vi "Main.vi"() -> ()   [LabVIEW 2025]
uses:
  State.ctl
  Replacement Channels.ctl
  NationalInstruments.VeriStand.SystemDefinitionAPI
panel:
  out "Array":T1[](array[typedef])
  out "Numeric":i32
  out "Deleted Channels":string[](array[string])
  in  "Delete Deprecated Channels":bool
  out "State":T2
  out "Replacement Log":string[](array[string])
  in  "stop":bool
  in  "Replace Signals":bool
  in  "Run Comparison Utility":bool
  in  "Available VCOM Signals (Replacement Channels)":string[](array[combo])=["CAN_Sender_Rx.ACC.ACC_ESP_E2E_PR2.ACC_ESP_E2E_PR2_CRC", "ESP_Rx.ACC.ACC_ESP_E2E_PR2.ACC_ESP_E2E_PR2_CRC", "CAN_Sender_Tx.ACC.NM_ACC.NM_ACC_ID", "ESP_Tx.ACC.NM_ACC.NM_ACC_ID"]
  in  "System Definition File Path":path=path "C:/dev/VCOM-SysDef-Utility/VCOM Config System Definition Utility/VeriStand Example Project/Example Project/Example Project.nivssdf"
  in  "Error in":errorcluster
  out "Signals Not Found in new VCOM Config (Channels to Replace)":string[](array[string])
  out "error out":errorcluster
  in  "VCOM config file in":path=path "C:/Users/Public/Documents/National Instruments/NI-VCOM/configuration/Single_Point/CAN/VCOMConfig.xml"
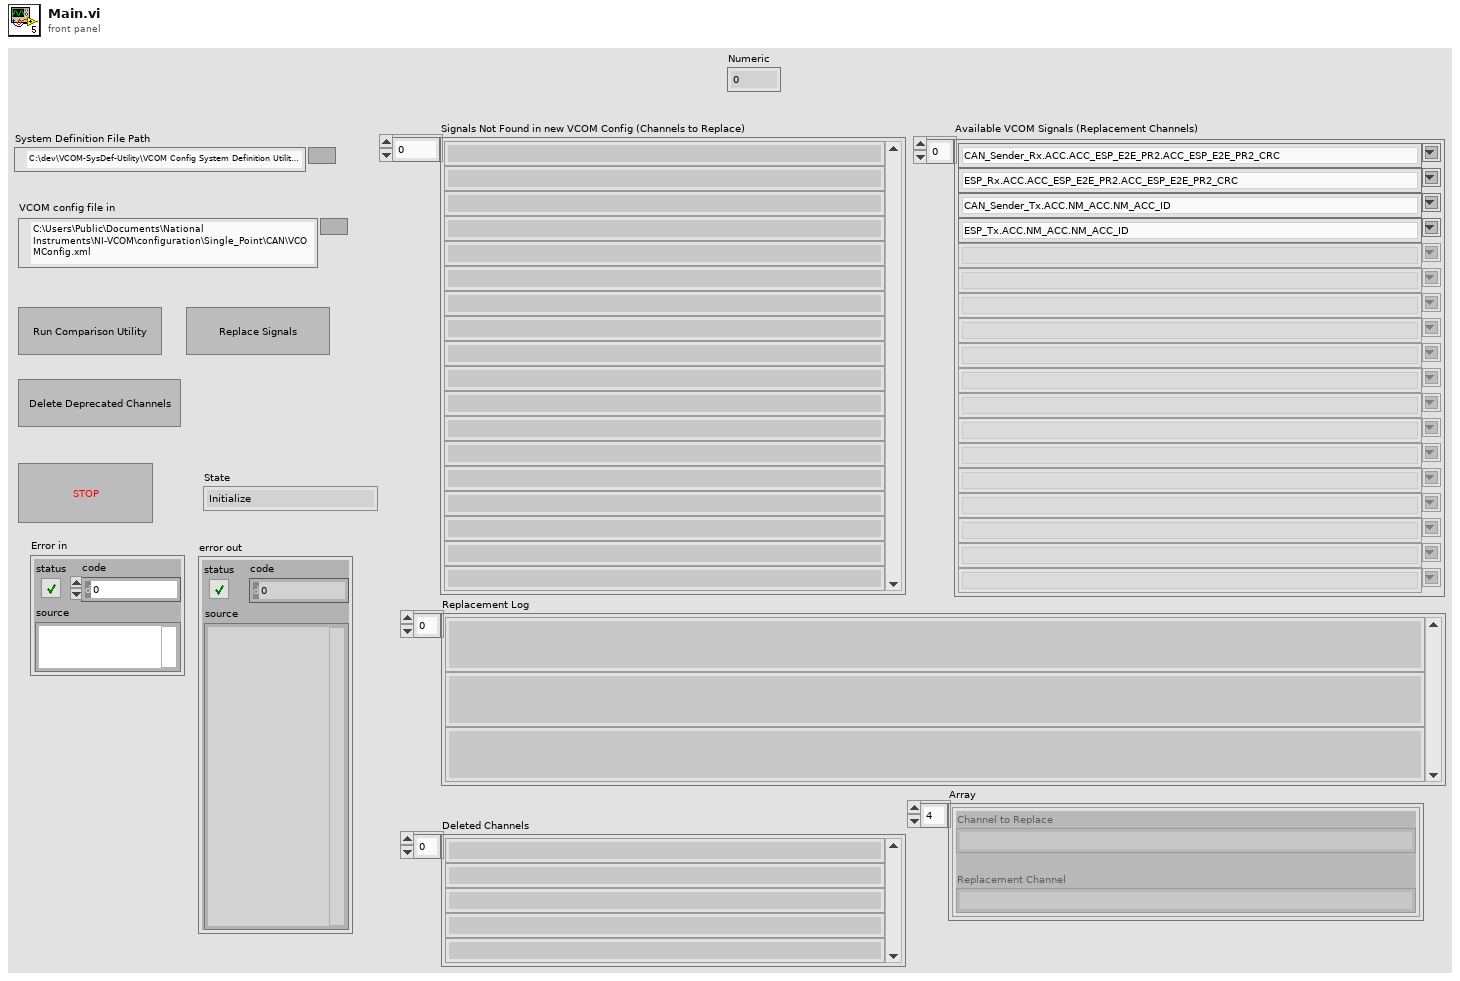
[diagram p1: front panel]
types:
  T1 = typedef "Replacement Channels.ctl" = cluster{"Channel to Replace":string, "Replacement Channel":string}
  T2 = typedef "State.ctl" = enum16{"Initialize", "Read VCOM Config", "Read System Definition", "Replace Signals", "Shutdown", "Wait for Event", "Delete Deprecated Channels"}
  T3 = typedef "Vehicle Communication Toolkit.lvlib/RBS Signal.ctl" = cluster{"Name":string, "Description":string, "Unit":string, "Lower Limit":dbl, "Upper Limit":dbl, "Signal Type":enum32{"RE_BOOL", "RE_UINT8", "RE_INT8", "RE_UINT16", "RE_INT16", "RE_UINT32", "RE_INT32", "RE_UINT64", "RE_INT64", "RE_FLOAT32", "RE_FLOAT64", "RE_TEXT"}, "Text Table":cluster{"Text":string, "Min":dbl, "Max":dbl}[], "ReadOnly":bool, "Signal Dimensions":u32[], "Default Value":dbl, "Code Page":u32}
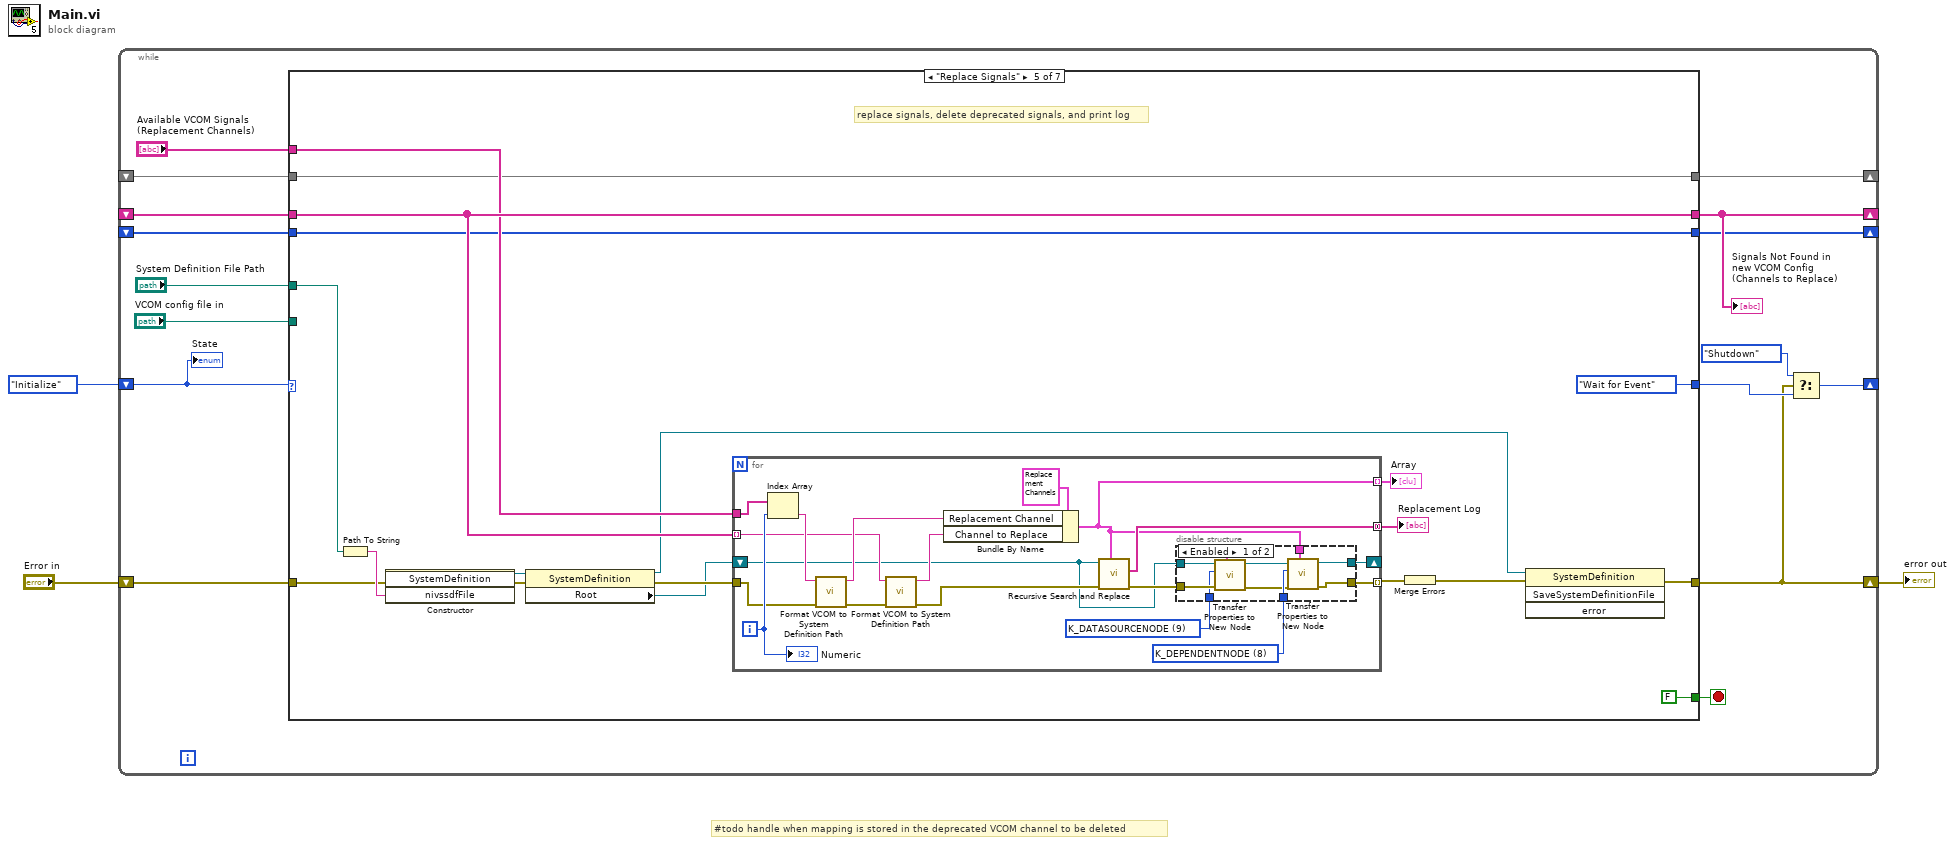
[diagram p0: block diagram]
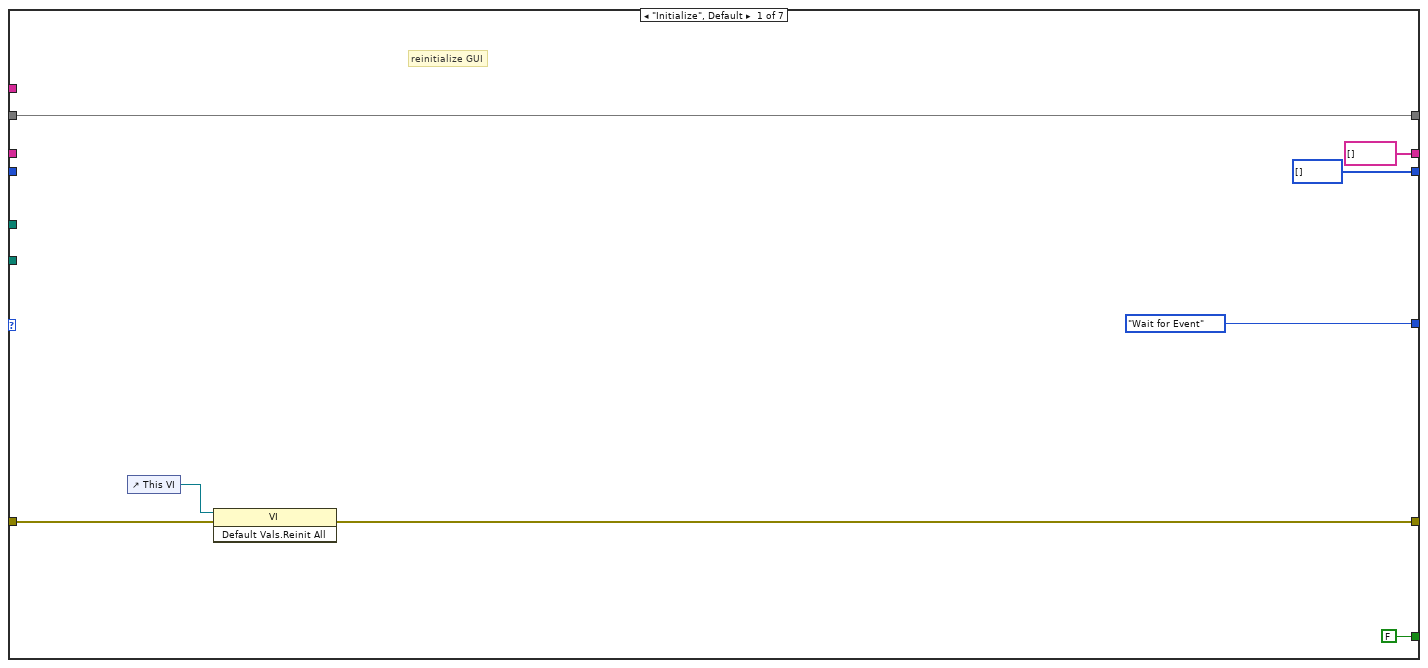
[diagram p2: hidden frame]
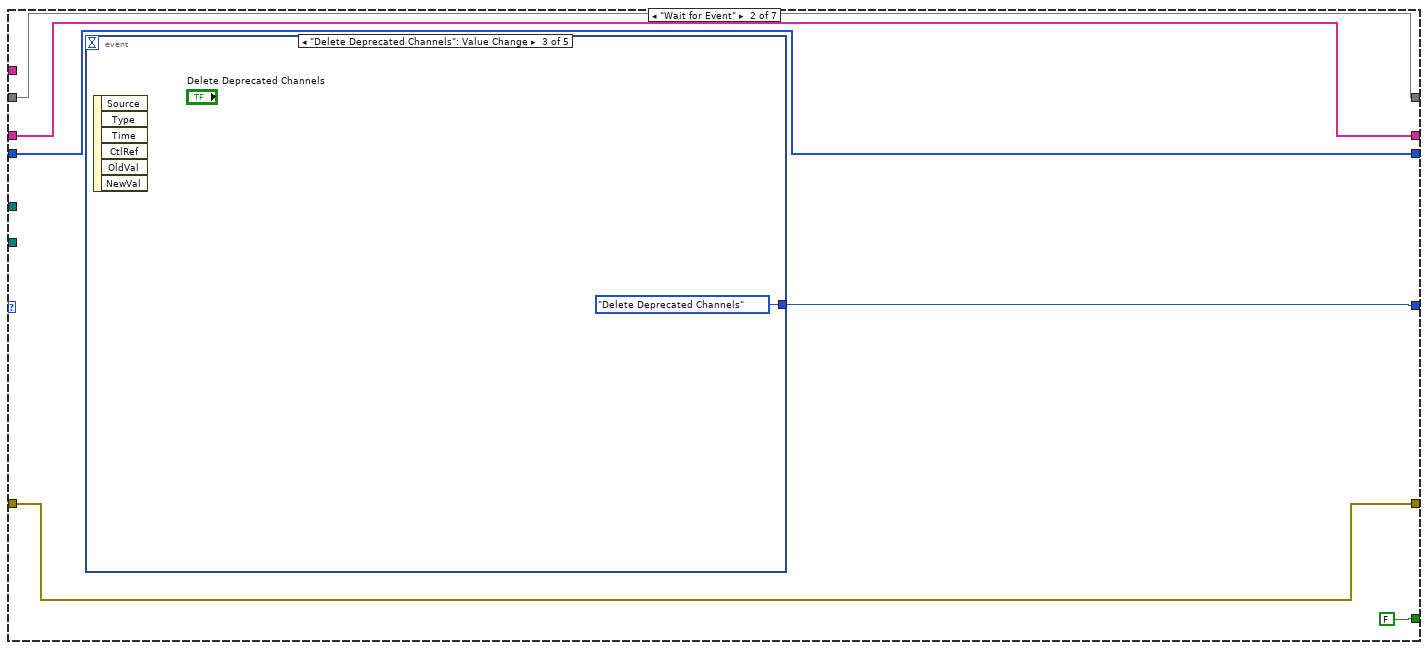
[diagram p3: hidden frame]
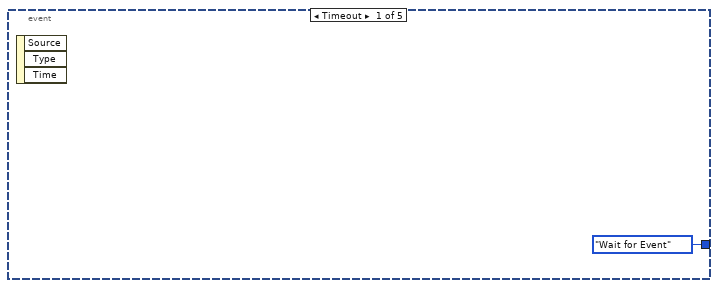
[diagram p4: hidden frame]
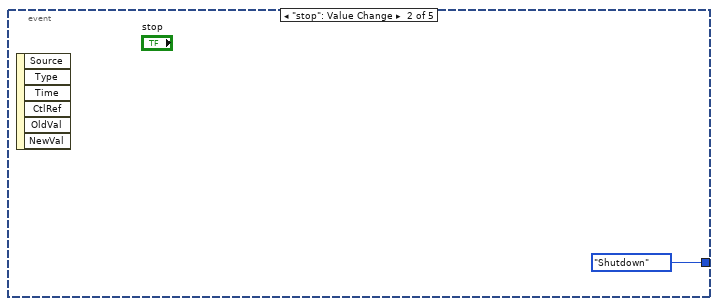
[diagram p5: hidden frame]
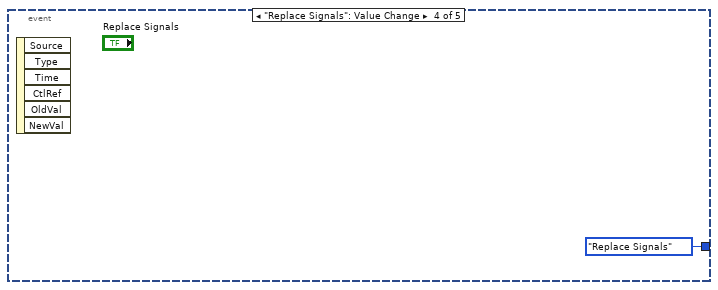
[diagram p6: hidden frame]
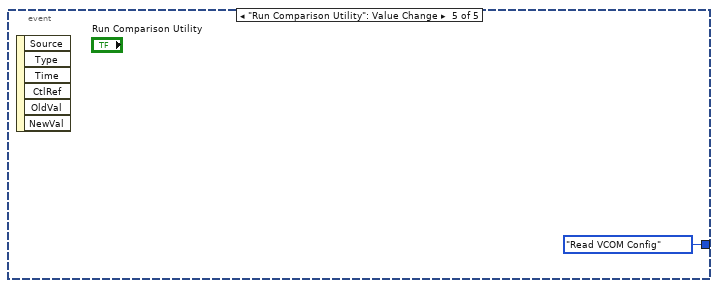
[diagram p7: hidden frame]
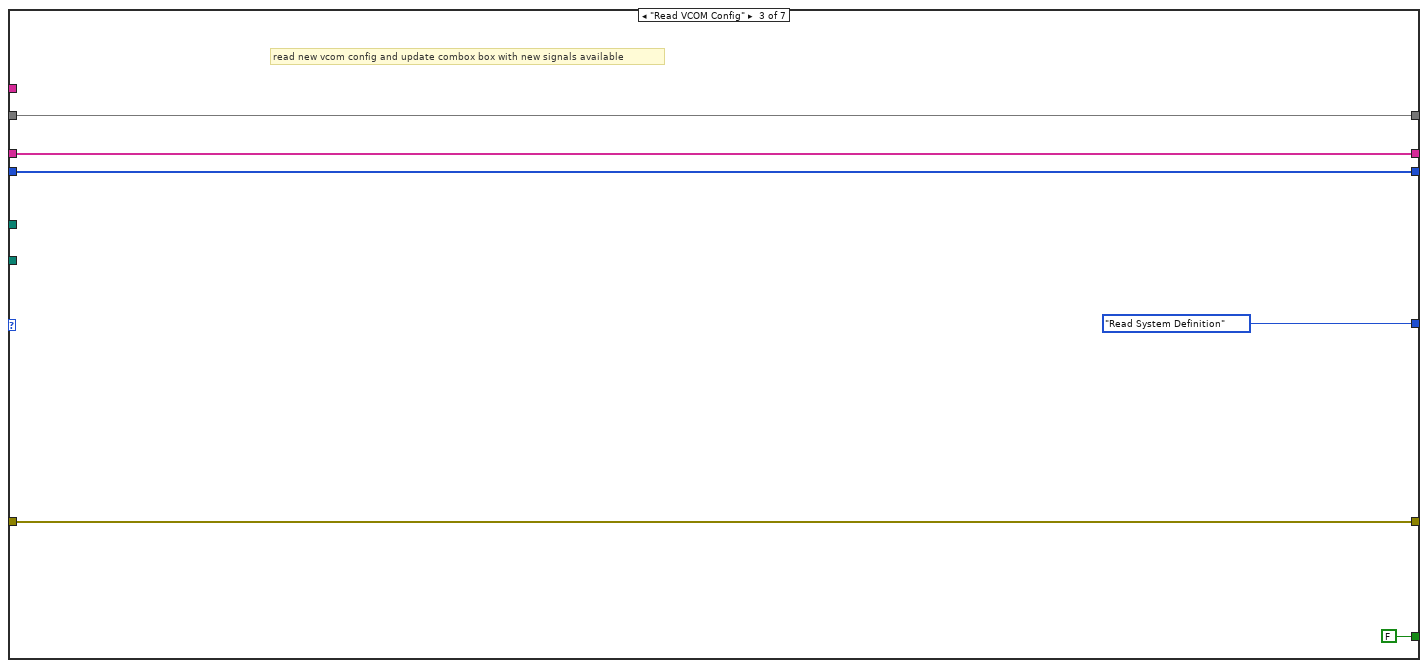
[diagram p8: hidden frame]
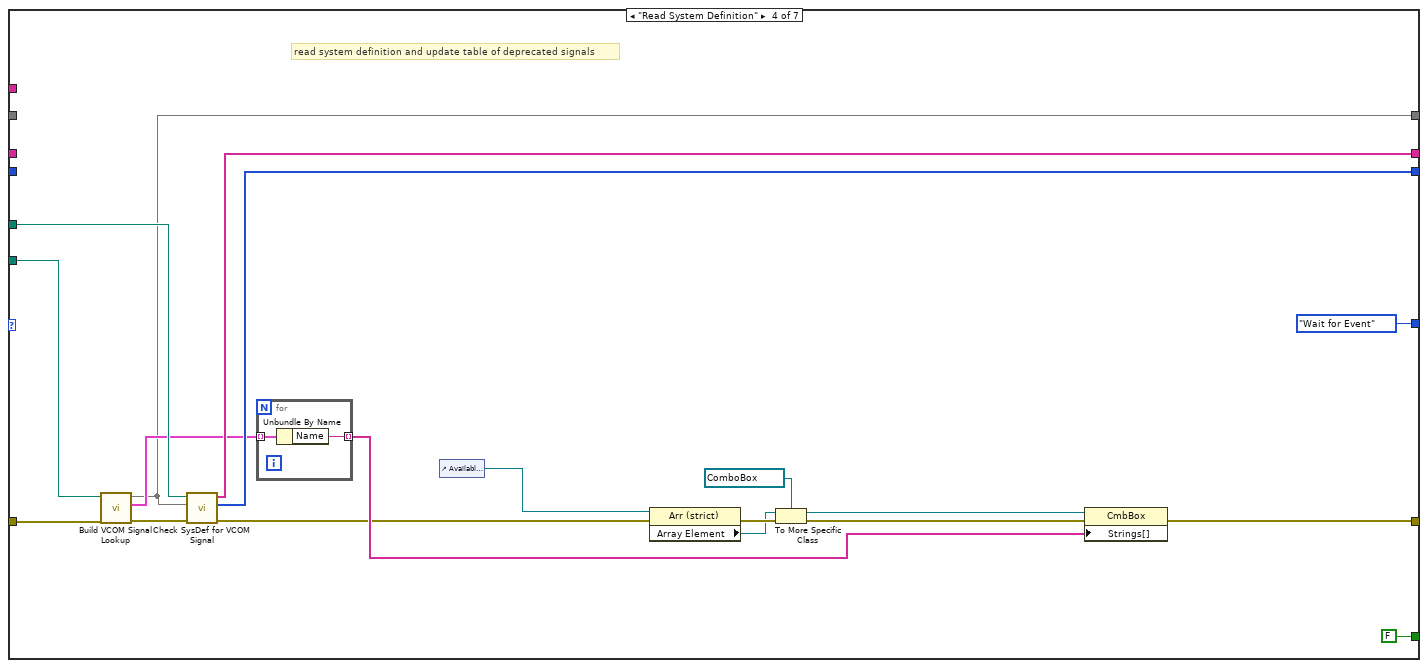
[diagram p9: hidden frame]
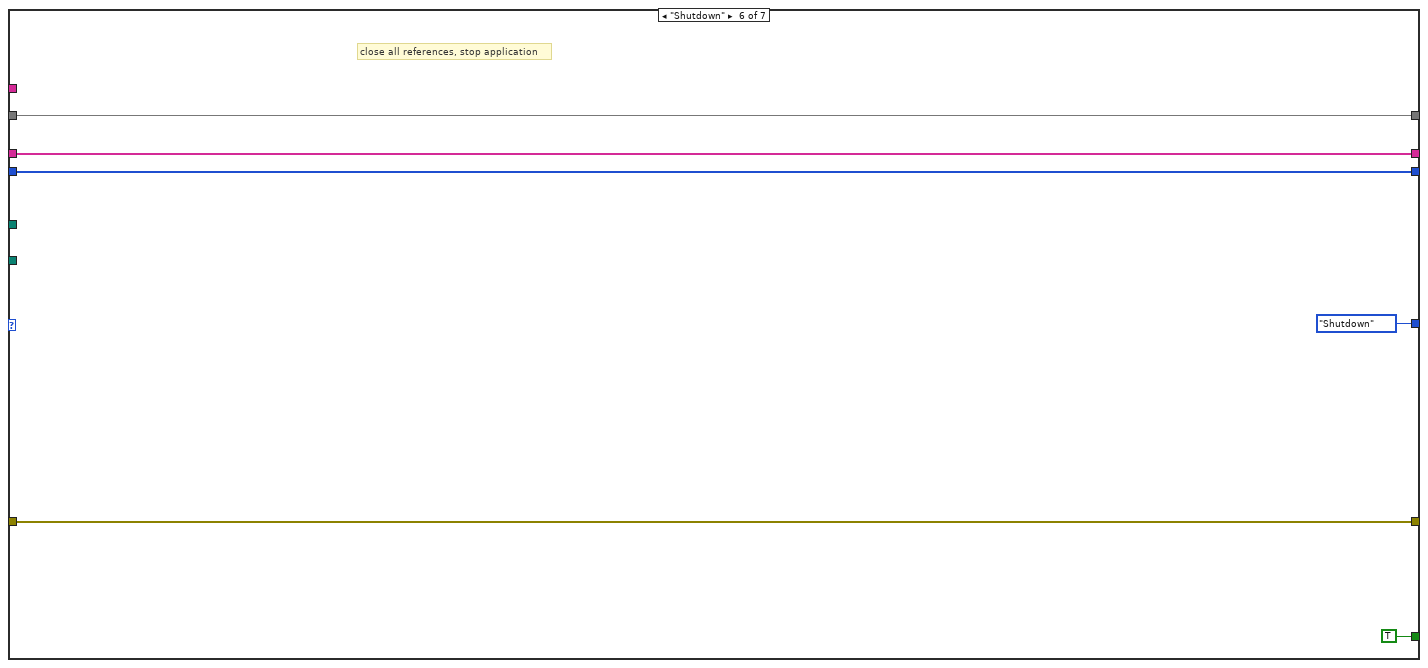
[diagram p11: hidden frame]
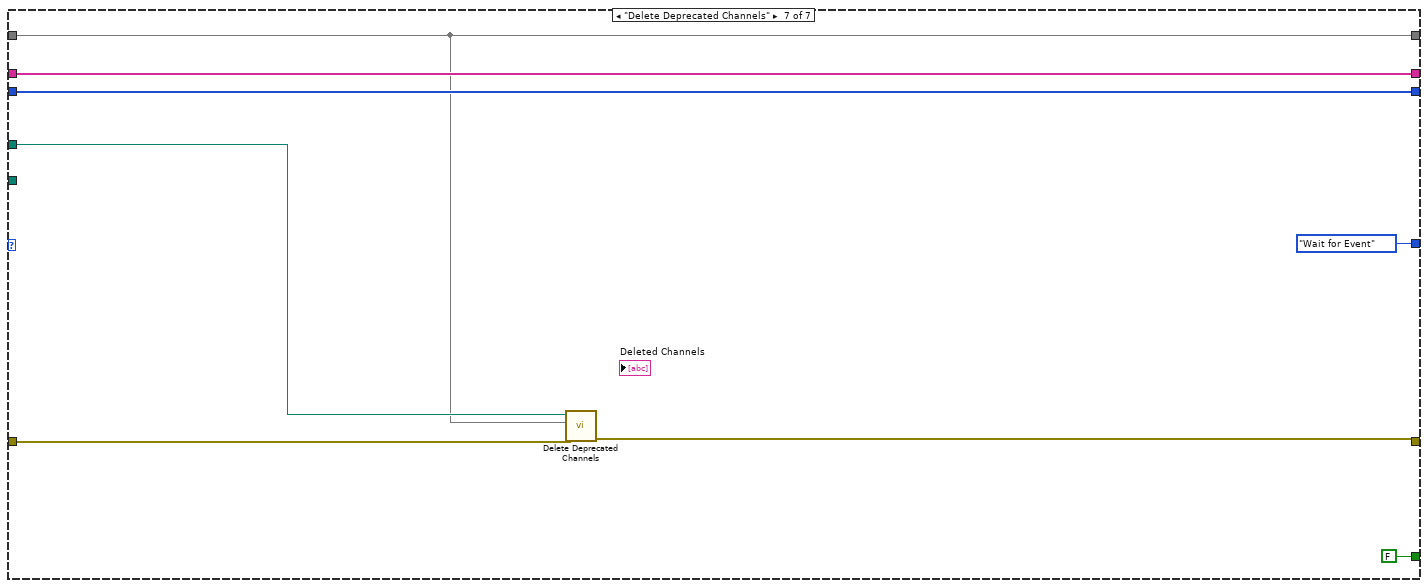
[diagram p12: hidden frame]
diagram:
  # "#todo handle when mapping is stored in the deprecated VCOM channel to be deleted"
  n1 = while {
    shift-right: [w15] -> _
    shift-left: State."Initialize" -> [w19]
    shift-right: [w11] -> _
    shift-left: _ -> [w10]
    shift-right: [w8] -> w1
    shift-left: "Error in" -> [w17]
    shift-right: [w7] -> _
    shift-left: _ -> [w6]
    shift-right: [w5] -> _
    shift-left: _ -> [w4]
    stop <- w18 stop-if-true
    n2 = case shown="\"Replace Signals\"" w19 {
      tunnel: [State."Wait for Event" w33 State."Read System Definition" State."Wait for Event" State."Wait for Event" State."Shutdown" State."Wait for Event"] -> w16
      tunnel: [FALSE FALSE FALSE FALSE FALSE TRUE FALSE] -> w18
      tunnel: [w24 w31 w43 w48 w72 w117 w122] -> w8
      tunnel: w17 -> [w25 w31 w43 w61 w81 w117 w124]
      tunnel: "VCOM config file in" -> [_ _ _ w59 _ _ _]
      tunnel: "System Definition File Path" -> [_ _ _ w58 w69 _ w123]
      tunnel: [string[] [] ("Signals Not Found in new VCOM Config") w30 w41 w57 w78 w116 w126] -> w11
      tunnel: w10 -> [_ w30 w41 _ w78 w116 w126]
      tunnel: "Available VCOM Signals (Replacement Channels)" -> [_ _ _ _ w77 _ _]
      tunnel: [u64[] [] ("Deprecated Signal GUIDs") w29 w40 w47 w71 w115 w121] -> w7
      tunnel: w6 -> [_ w29 w40 _ w71 w115 w121]
      tunnel: [w20 w28 w39 w45 w70 w114 w120] -> w5
      tunnel: w4 -> [w20 w28 w39 _ w70 w114 w120]
      frame "Initialize", Default {
        # "reinitialize GUI"
        n3 = control-ref of="This VI"() -> (w26:refnum<vi>)
        n4 = invoke class="VI" method="Default Vals.Reinit All"(reference=w26, error in=w25) -> (error out=w24:errorcluster)  [unwired: 1 in, 2 out]
      }
      frame "Wait for Event" {
        n5 = event shown="[2] \"Delete Deprecated Channels\": Value Change" {
          selector: _ -> [_ _ _ _ _]
          dyn-events: _ -> [_ _ _ _ _]
          timeout: _ -> [_ _ _ _ _]
          tunnel: [State."Wait for Event" State."Shutdown" State."Delete Deprecated Channels" State."Replace Signals" State."Read VCOM Config"] -> w33
          event Timeout {
            n6 = event-data() -> ()  [unwired: 1 in, 3 out]
          }
          event "stop": Value Change {
            n7 = event-data() -> ()  [unwired: 1 in, 6 out]
          }
          event "Delete Deprecated Channels": Value Change {
            n8 = event-data() -> ()  [unwired: 1 in, 6 out]
          }
          event "Replace Signals": Value Change {
            n9 = event-data() -> ()  [unwired: 1 in, 6 out]
          }
          event "Run Comparison Utility": Value Change {
            n10 = event-data() -> ()  [unwired: 1 in, 6 out]
          }
        }
      }
      frame "Read VCOM Config" {
        # "read new vcom config and update combox box with new signals available"
      }
      frame "Read System Definition" {
        # "read system definition and update table of deprecated signals"
        n11 = call "Build VCOM Signal Lookup.vi"("Error in"=w61, "VCOM config file in"=w59) -> ("Error out"=w60:errorcluster, "VCOM signal list"=w46:T3[], "VCOM Signal Map"=w45:map{string, T3})  [unwired: 7 in]
        n12 = call "Check SysDef for VCOM Signal.vi"("error in (no error)"=w60, "VCOM Signal Map In"=w45, "System Definition File Path"=w58) -> ("error out"=w50:errorcluster, "Deprecated Signal GUIDs"=w47:u64[], "Signals Not Found in new VCOM Config"=w57:string[])  [unwired: 6 in]
        n13 = for {
          tunnel: w46 -> [w65] mode=indexing
          tunnel: [w64] -> w52 mode=indexing
          n14 = Unbundle By Name(w65) -> ("Name"=w64:string)
        }
        n15 = control-ref of="Available VCOM Signals (Replacement Channels)"() -> (w51:refnum<vi>)
        n16 = property class="Arr (strict)"(reference=w51, error in=w50) -> (error out=w56:errorcluster, "Array Element"=w55:refnum<vi>)  [unwired: 1 out]
        n17 = To More Specific Class(target class=refnum<vi> refnum ("Combo Box"), reference=w55, error in=w56) -> (specific class reference=w54:refnum<vi>, error out=w49:errorcluster)
        n18 = property class="CmbBox"(reference=w54, error in=w49, "Strings[]"=w52) -> (error out=w48:errorcluster)  [unwired: 1 out]
      }
      frame "Replace Signals" {
        # "replace signals, delete deprecated signals, and print log"
        n19 = Path To String(path=w69) -> (string=w83:string)
        n20 = constructor class="SystemDefinition"(error in=w81, "nivssdfFile"=w83) -> (reference out=w79:refnum<k24>, error out=w82:errorcluster)  [unwired: 2 in, 2 out]
        n21 = property class="SystemDefinition"(reference=w79, error in=w82) -> (reference out=w68:refnum<k24>, error out=w80:errorcluster, "Root"=w67:refnum<k24>)
        n22 = for {
          tunnel: w80 -> [w98]
          tunnel: w78 -> [w93] mode=indexing
          tunnel: w77 -> [w100]
          tunnel: [w89] -> w76 mode=indexing
          tunnel: [w99] -> w75 mode=concatenating
          shift-right: [w87] -> _
          shift-left: w67 -> [w86]
          tunnel: [w85] -> w66 mode=indexing
          i -> [w101]
          w88 = 8 items=["K_STRING", "K_BOOL", "K_I32", "K_U32", "K_DOUBLE", "K_U64", "K_VARIANT", "K_DEPENDENTFILE", "K_DEPENDENTNODE", "K_DATASOURCENODE", "K_U16", "K_DBLARR", "K_U32ARR", "K_I32ARR", "K_STRINGARR", "K_DICTIONARY", "K_DICTIONARYARR", "K_BINARYSTRING", "K_I16", "K_I64", "K_BOOLARR", "K_U64ARR", "K_U16ARR", "K_I64ARR", "K_I16ARR"] ("Property Type")
          w90 = 9 items=["K_STRING", "K_BOOL", "K_I32", "K_U32", "K_DOUBLE", "K_U64", "K_VARIANT", "K_DEPENDENTFILE", "K_DEPENDENTNODE", "K_DATASOURCENODE", "K_U16", "K_DBLARR", "K_U32ARR", "K_I32ARR", "K_STRINGARR", "K_DICTIONARY", "K_DICTIONARYARR", "K_BINARYSTRING", "K_I16", "K_I64", "K_BOOLARR", "K_U64ARR", "K_U16ARR", "K_I64ARR", "K_I16ARR"] ("Property Type")
          n23 = Index Array(array=w100, index=w101) -> (element=w95:string)
          n24 = call "Format VCOM to System Definition Path.vi"("error in (no error)"=w98, "VCOM Signal"=w95) -> ("error out"=w97:errorcluster, "System Definition Path"=w94:string)  [unwired: 8 in]
          n25 = call "Format VCOM to System Definition Path.vi"("error in (no error)"=w97, "VCOM Signal"=w93) -> ("error out"=w96:errorcluster, "System Definition Path"=w92:string)  [unwired: 8 in]
          n26 = Bundle By Name(cluster=T1 {"Channel to Replace"="Targets/Controller/Custom Devices/VCOM/CAN_Sender_Tx/ACC/ACC_ESP_E2E_PR2/ACC_NEW_SIGNAL", "Replacement Channel"="Targets/Controller/User Channels/User Channel 1"} ("Replacement Channels"), "Replacement Channel"=w94, "Channel to Replace"=w92) -> (w85:T1)
          n27 = call "Recursive Search and Replace.vi"("Replacement Channels"=w85, "error in (no error)"=w96, ".NET Refnum"=w86) -> ("error out"=w91:errorcluster, "Replacement Log"=w99:string[])  [unwired: 7 in]
          n28 = disable-structure shown="Enabled" {
            disable-tunnel: w91 -> [w111 w113]
            disable-tunnel: w90 -> [w110 _]
            disable-tunnel: [w109 w113] -> w89
            disable-tunnel: w85 -> [w108 _]
            disable-tunnel: w88 -> [w107 _]
            disable-tunnel: [w104 w112] -> w87
            disable-tunnel: w86 -> [w103 w112]
            frame Enabled {
              n29 = call "Transfer Properties to New Node.vi"("Replacement Channels"=w108, "error in (no error)"=w111, "Property Type"=w110, "reference"=w103) -> ("error out"=w106:errorcluster, "reference out"=w105:refnum<k24>)  [unwired: 5 in, 1 out]
              n30 = call "Transfer Properties to New Node.vi"("Replacement Channels"=w108, "error in (no error)"=w106, "Property Type"=w107, "reference"=w105) -> ("error out"=w109:errorcluster, "reference out"=w104:refnum<k24>)  [unwired: 5 in, 1 out]
            }
            frame Disabled {
            }
          }
          "Numeric" <- w101
        }
        "Replacement Log" <- w75
        "Array" <- w66
        n31 = Merge Errors(w76) -> (w73:errorcluster)
        n32 = invoke class="SystemDefinition" method="SaveSystemDefinitionFile"(reference=w68, error in=w73) -> (error out=w72:errorcluster)  [unwired: 2 in, 3 out]
      }
      frame "Shutdown" {
        # "close all references, stop application"
      }
      frame "Delete Deprecated Channels" {
        n33 = call "Delete Deprecated Channels.vi"("error in (no error)"=w124, "VCOM Signal Map In"=w120, "System Definition File Path"=w123) -> ("error out"=w122:errorcluster)  [unwired: 8 in]
      }
    }
    "Signals Not Found in new VCOM Config (Channels to Replace)" <- w11
    n34 = Select(t=State."Shutdown", s=w8, f=w16) -> (s? t:f=w15:T2)
    "State" <- w19
  }
  "error out" <- w1
